vi "Get Value (Boolean).vi"(8 "error in (no error)":errorcluster, 10 "Name":string, 11 "Camera in":refnum<class "Camera.lvclass">) -> (0 "error out":errorcluster, 2 "Value":bool, 3 "Camera":refnum<class "Camera.lvclass">)   [LabVIEW 2020, in "Camera.lvclass"]
uses:
  Camera.lvclass
  Camera.lvclass/Camera.ctl
  Check Not Disconnected.vi
  <vilib>/Utility/error.llb/Error Cluster From Error Code.vi
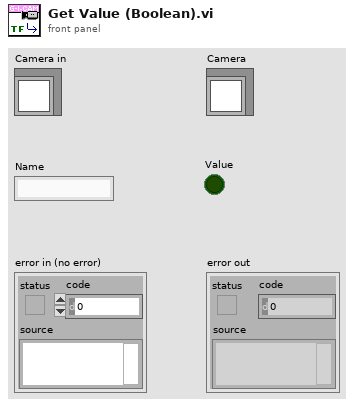
[diagram p1: front panel]
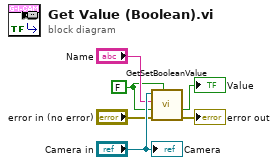
[diagram p0: block diagram]
diagram:
  w1 = FALSE ("Set?")
  n1 = call "GetSetBooleanValue.vi"("Set?"=w1, "error in (no error)"="error in (no error)", "Value In"=w1, "Name"="Name", "Camera in"="Camera in") -> ("error out"=→"error out":errorcluster, "Value Out"=→"Value":bool)  [unwired: 5 in]
  "Camera" <- "Camera in"
